vi "HMI.vi"(8 "error in (no error)":errorcluster caption="entrée d'erreur (pas d'erreur)", 11 "Class Popup Autotest (Default) en entrée":refnum<class "Popup Autotest (Default).lvclass">) -> (0 "error out":errorcluster caption="sortie d'erreur", 1 "Input":string, 2 "Autotest":bool, 3 "Class Popup Autotest (Default) en sortie":refnum<class "Popup Autotest (Default).lvclass">)   [LabVIEW 2020, in "Library Instrument & Equipement.lvlib" / "Library Popup.lvlib" / "Popup Autotest (Default).lvclass"]
uses:
  Popup Autotest (Default).lvclass
  Commun VI/TypeDef/Commande Popup autotest/Commande element autotest.ctl
  Class Popup (Main)/Class Popup (Main).lvclass
panel:
  out "Element test":T2
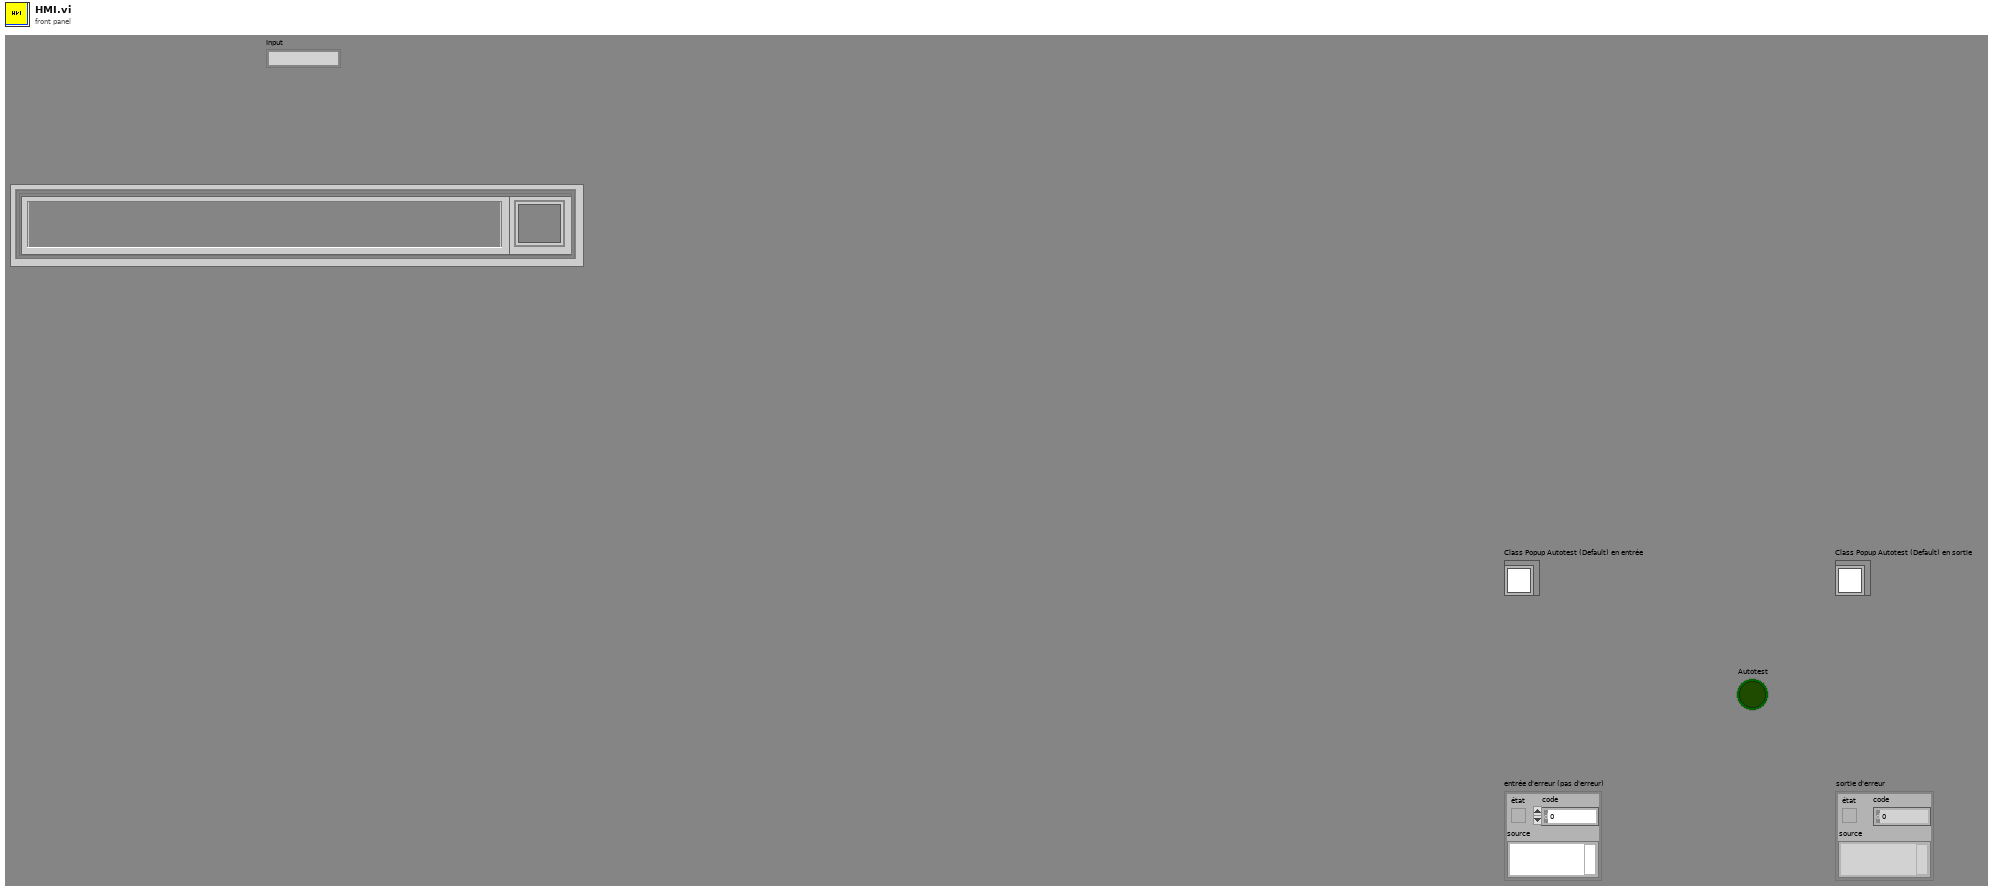
[diagram p1: front panel]
types:
  T1 = typedef "Commande element autotest.ctl" = cluster{"Instrument":string, "Etat":cluster{"Menu déroulant":u16}}
  T2 = cluster{"Element autotest":T1, "Element autotest 2":T1, "Element autotest 3":T1, "Element autotest 4":T1, "Element autotest 5":T1, "Element autotest 6":T1, "Element autotest 7":T1, "Element autotest 8":T1, "Element autotest 9":T1}
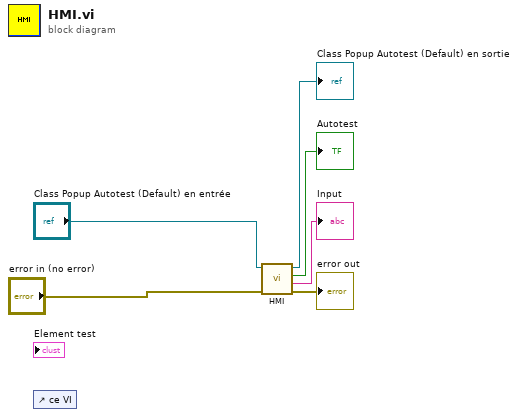
[diagram p0: block diagram]
diagram:
  n1 = control-ref of="ce VI"() -> ()  [unwired: 1 out]
  n2 = call-parent "HMI.vi"("error in (no error)"="error in (no error)", "Class Popup (Main) en entrée"="Class Popup Autotest (Default) en entrée") -> ("error out"=→"error out":errorcluster, "Input"=→"Input":string, "Operator_Selection"=→"Autotest":bool, "Class Popup (Main) en sortie"=→"Class Popup Autotest (Default) en sortie":refnum<class "Popup Autotest (Default).lvclass">)  [unwired: 6 in]
